vi "Set VI Properties for Debugging Mode.vi"(8 "error in":errorcluster, 10 "Debug mode?":bool, 11 "Launcher VI ref":refnum<vi>) -> (0 "error out":errorcluster, 3 "Launcher VI ref out":refnum<vi>)   [LabVIEW 2020, in "Launcher Support.lvlib"]
doc: "This VI sets the properties of the VI Launcher to either headless or debugging mode.\n_____\nBased on DQMH Project Template 7.0.1.1316."
uses:
  Launcher Support.lvlib
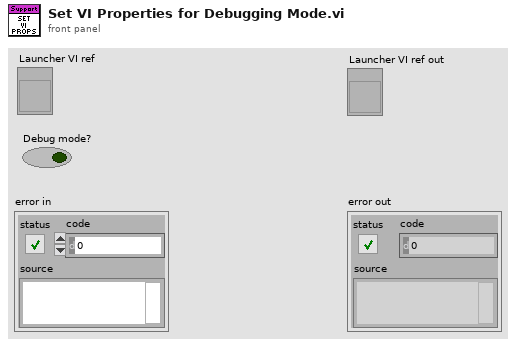
[diagram p1: front panel]
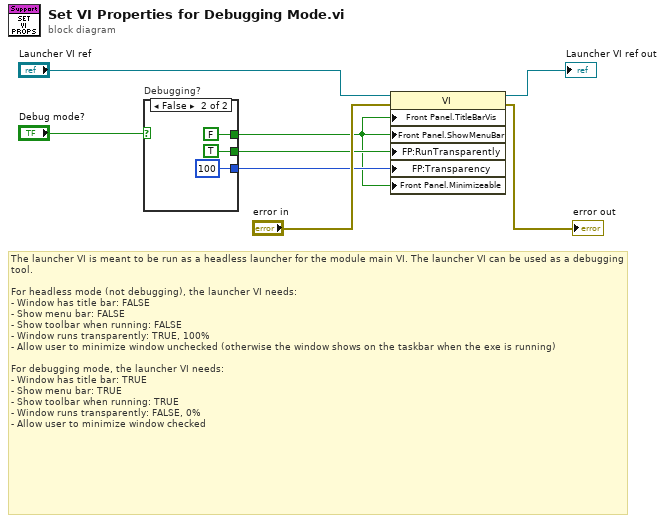
[diagram p0: block diagram]
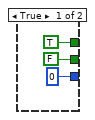
[diagram p2: hidden frame]
diagram:
  # "The launcher VI is meant to be run as a headless launcher for the module main VI. The launcher VI can be used as a debugging tool.\n\nFor headless mode (not debugging), the launcher VI needs:\n- Window has title bar: FALSE\n- Show menu bar: FALSE\n- Show toolbar when running: FALSE\n- Window runs transparently: TRUE, 100%\n- Allow user to minimize window unchecked (otherwise the window shows on the taskbar when the exe is running)\n\nFor debugging mode, the launcher VI needs:\n- Window has title bar: TRUE\n- Show menu bar: TRUE\n- Show toolbar when running: TRUE\n- Window runs transparently: FALSE, 0%\n- Allow user to minimize window checked"
  n1 = case "Debugging?" shown="False" "Debug mode?" {
    tunnel: [TRUE FALSE] -> w4
    tunnel: [FALSE TRUE] -> w6
    tunnel: [u8 0 ("Front Panel Window:Transparency") u8 100 ("Front Panel Window:Transparency")] -> w5
    frame True {
    }
    frame False {
    }
  }
  n2 = property class="VI"(reference="Launcher VI ref", error in="error in", "Front Panel.TitleBarVis"=w4, "Front Panel.ShowMenuBar"=w4, "FP:RunTransparently"=w6, "FP:Transparency"=w5, "Front Panel.Minimizeable"=w4) -> (reference out=→"Launcher VI ref out":refnum<vi>, error out=→"error out":errorcluster)
